vi "CAN Log Queue FGV Release the Reference.vi"(8 "error in":errorcluster, 11 "Selected Sockets":i16[](array[numeric])) -> (0 "error out":errorcluster)   [LabVIEW 2023, in "LTT_TeststandSteptypes.lvlib"]
uses:
  LTT_TeststandSteptypes.lvlib
  Control/CAN FGV State.ctl
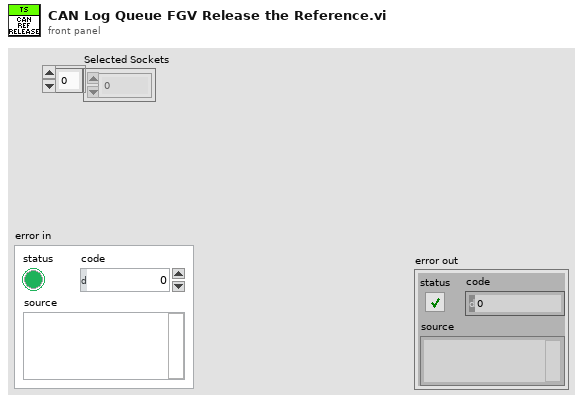
[diagram p1: front panel]
types:
  T1 = typedef "LTT_TeststandSteptypes.lvlib/CAN FGV State.ctl" = enum16{"Init", "Get", "Set"}
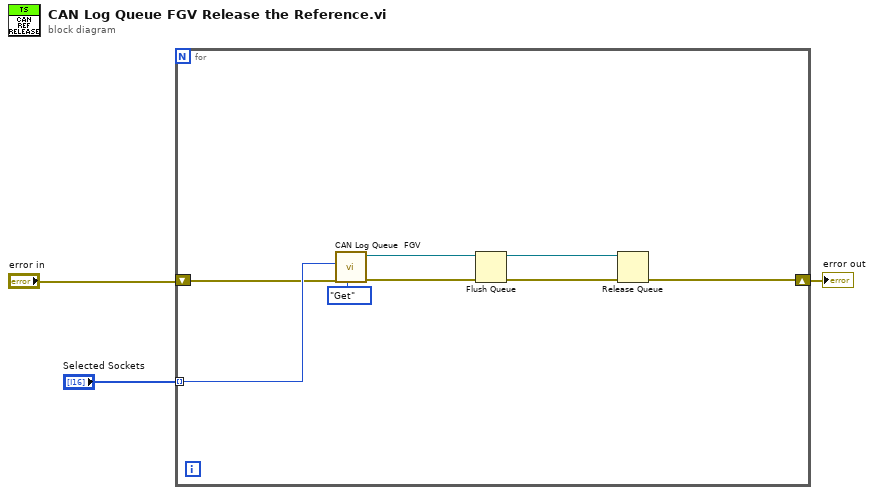
[diagram p0: block diagram]
diagram:
  n1 = for {
    tunnel: "Selected Sockets" -> [w10] mode=indexing
    shift-right: [w5] -> w1
    shift-left: "error in" -> [w9]
    n2 = call "CAN Log Queue  FGV.vi"("CAN FGV State"=CAN_FGV_State."Get", "error in"=w9, "Current Scoket"=w10) -> ("error out"=w8:errorcluster, "Log queue out"=w7:refnum<queue>)  [unwired: 7 in]
    n3 = Flush Queue(queue=w7, error in (no error)=w8) -> (queue out=w4:refnum<queue>, error out=w6:errorcluster)  [unwired: 1 out]
    n4 = Release Queue(queue=w4, error in (no error)=w6) -> (error out=w5:errorcluster)  [unwired: 1 in, 2 out]
  }
  "error out" <- w1
